vi "hour_txt.vi"() -> ()   [LabVIEW 2017]
panel:
  in  "hour_txt":dbl
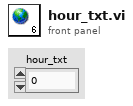
[diagram p1: front panel]
diagram:
